vi "Cache.DUT.Read.vi"(8 "error in (no error)":errorcluster, 11 "ResultsPath":path=path "D:/svn/LineTraceSystem/SOFTWARE/logs/results") -> (0 "error out":errorcluster, 1 "Groups":i32[](array[numeric]), 2 "Results out":T1[](array[typedef]))   [LabVIEW 2016]
uses:
  Cache.TestSteps.Fglb.ResultData.ctl
  Database/ProdaNG/Controls/ProdaNG.ProcessResult.ctl
  Database/ProdaNG/Controls/ProdaNG.ProcessStepResult.ctl
  Database/ProdaNG/Controls/ProdaNG.TestStepResult.ctl
  Database/ProdaNG/Controls/ProdaNG.TestValueResult.ctl
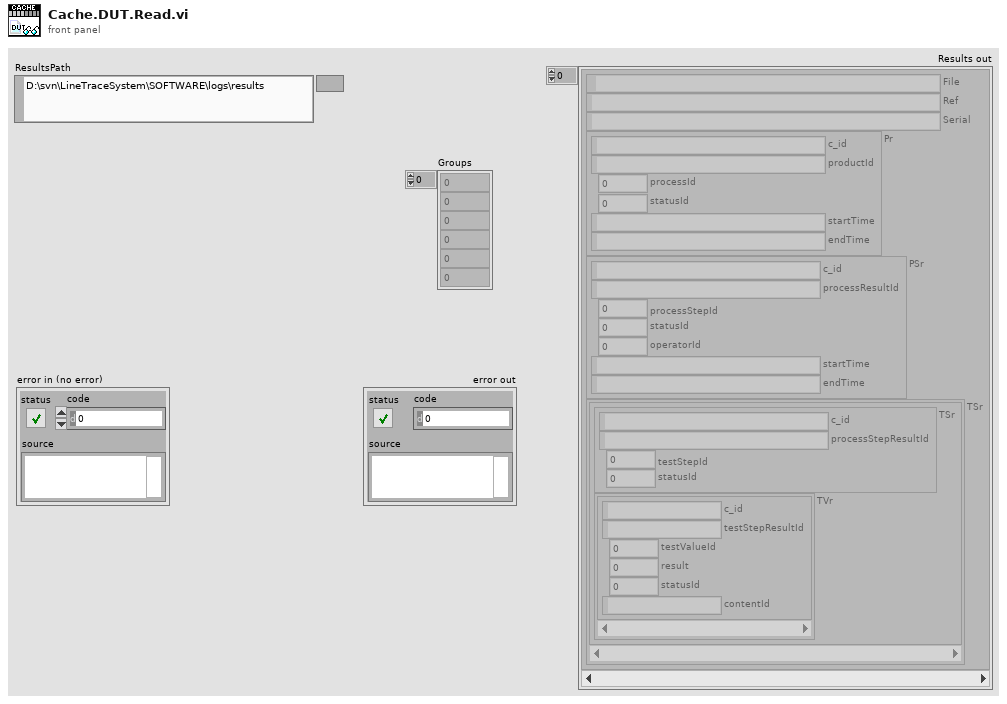
[diagram p1: front panel]
types:
  T1 = typedef "Cache.TestSteps.Fglb.ResultData.ctl" = cluster{"File":path, "Ref":string, "Serial":string, "Pr":T2, "PSr":T3, "TSr":cluster{"TSr":T4, "TVr":T5[]}[]}
  T2 = typedef "ProdaNG.ProcessResult.ctl" = cluster{"c_id":string, "productId":string, "processId":i32, "statusId":i32, "startTime":string, "endTime":string}
  T3 = typedef "ProdaNG.ProcessStepResult.ctl" = cluster{"c_id":string, "processResultId":string, "processStepId":i32, "statusId":i32, "operatorId":i32, "startTime":string, "endTime":string}
  T4 = typedef "ProdaNG.TestStepResult.ctl" = cluster{"c_id":string, "processStepResultId":string, "testStepId":i32, "statusId":i32}
  T5 = typedef "ProdaNG.TestValueResult.ctl" = cluster{"c_id":string, "testStepResultId":string, "testValueId":i32, "result":dbl, "statusId":i32, "contentId":string}
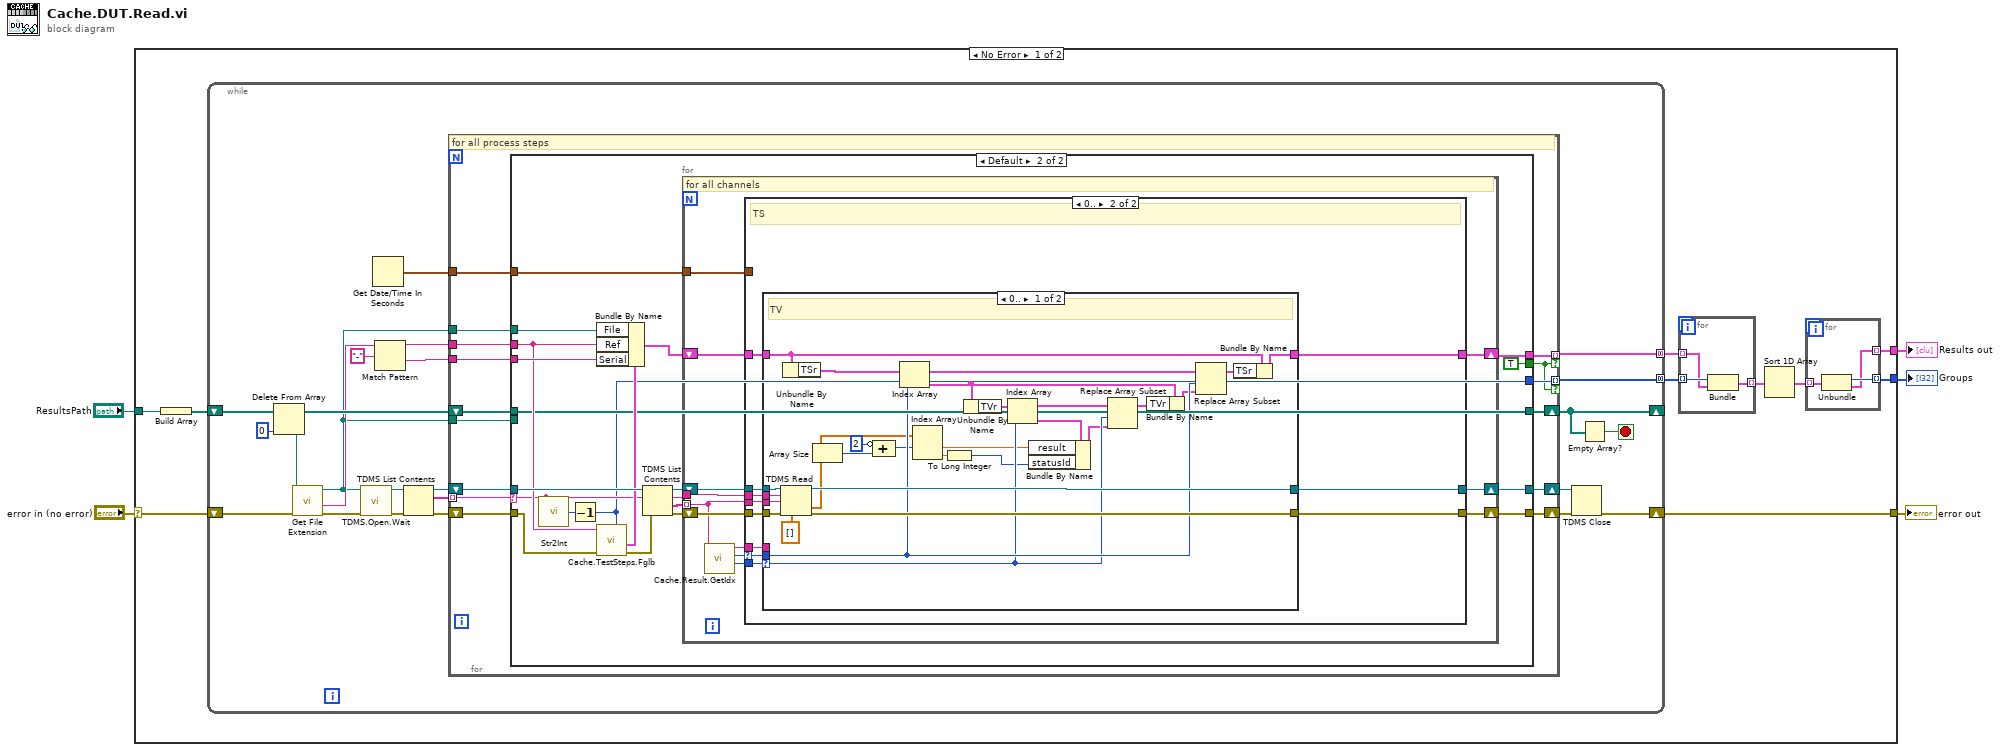
[diagram p0: block diagram]
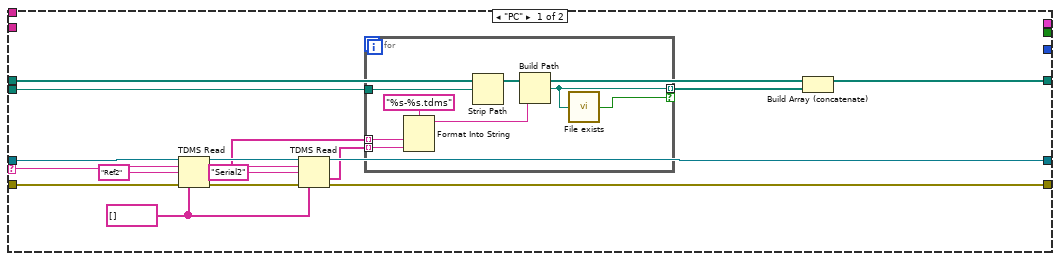
[diagram p2: hidden frame]
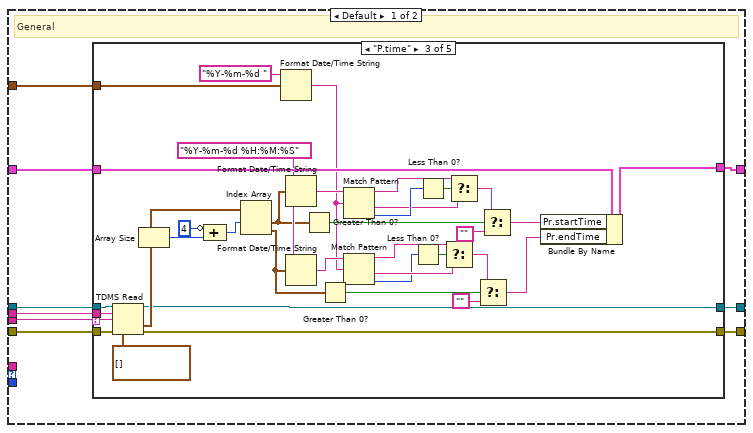
[diagram p3: hidden frame]
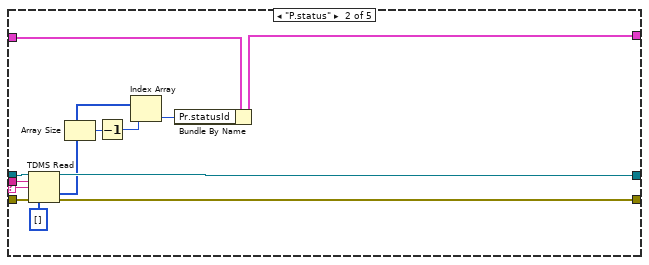
[diagram p5: hidden frame]
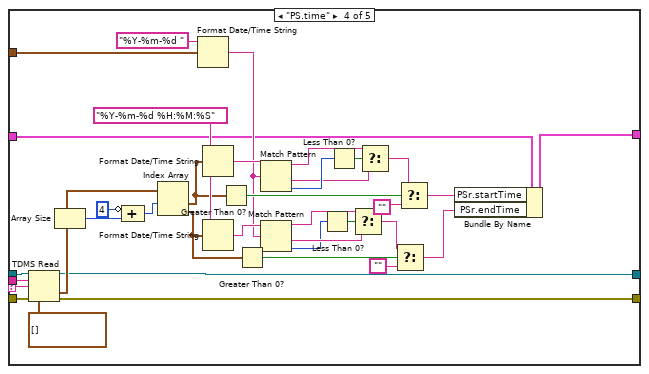
[diagram p6: hidden frame]
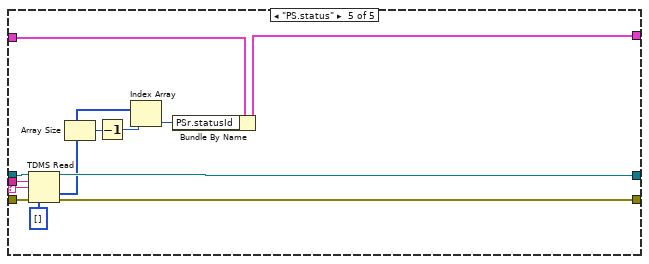
[diagram p7: hidden frame]
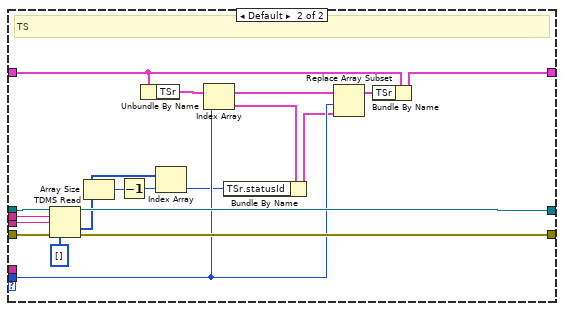
[diagram p8: hidden frame]
diagram:
  n1 = case shown="No Error" "error in (no error)" {
    selector: "error in (no error)" -> [w14 w286]
    tunnel: [w15 w286] -> w5
    tunnel: "ResultsPath" -> [w13 _]
    tunnel: [w6 _] -> w2
    tunnel: [w7 _] -> w1
    frame No Error {
      n2 = Build Array(w13) -> (w12:path[])
      n3 = while {
        tunnel: [w44] -> w11 mode=concatenating
        tunnel: [w42] -> w10 mode=concatenating
        shift-right: [w45] -> w15
        shift-left: w14 -> [w43]
        shift-right: [w25] -> _
        shift-left: w12 -> [w41]
        stop <- w24 stop-if-true
        n4 = Delete From Array(array=w41, index=0) -> (deleted portion=w27:path, array with subset deleted=w26:path[])  [unwired: 1 in]
        n5 = call <vilib>:"Get File Extension.vi"("error in (no error)"=w43, "file"=w27) -> ("error out"=w35:errorcluster, "filename without extension"=w23:string, "dup file"=w22:path)  [unwired: 5 in, 2 out]
        n6 = call "TDMS.Open.Wait.vi"("error in (no error)"=w35, "file path"=w22) -> ("error out"=w31:errorcluster, "tdms file out"=w38:refnum<k34>)  [unwired: 8 in]
        n7 = Get Date/Time In Seconds() -> (seconds since 1Jan1904=w29:timestamp)
        n8 = Match Pattern(string=w23, regular expression="-") -> (before substring=w33:string, after substring=w32:string)  [unwired: 1 in, 2 out]
        n9 = TDMS List Contents(4:w31, 7:w38) -> (0:w39:errorcluster, 2:w30:string[], 3:w40:refnum<k34>)  [unwired: 1 in, 1 out]
        n10 = for {
          shift-right: [w60] -> w37
          shift-left: w39 -> [w55]
          shift-right: [w59] -> w36
          shift-left: w40 -> [w57]
          tunnel: w30 -> [w52] mode=indexing
          tunnel: [w58] -> w44 mode=indexing if=w47
          tunnel: w33 -> [w54]
          tunnel: w32 -> [w56]
          tunnel: w29 -> [w53]
          tunnel: w22 -> [w51]
          shift-right: [w49] -> w25
          shift-left: w26 -> [w50]
          tunnel: [w48] -> w42 mode=indexing if=w47
          tunnel: w22 -> [w46]
          # "for all process steps"
          n11 = case shown="Default" w52 {
            selector: w52 -> [w75 w89]
            tunnel: [w68 w106] -> w60
            tunnel: [w67 w105] -> w59
            tunnel: [_ w104] -> w58
            tunnel: w57 -> [w76 w102]
            tunnel: w56 -> [_ w96]
            tunnel: w55 -> [w77 w95]
            tunnel: w54 -> [_ w94]
            tunnel: w53 -> [_ w93]
            tunnel: w51 -> [w66 _]
            tunnel: [_ TRUE] -> w47
            tunnel: w50 -> [w62 w90]
            tunnel: [w61 w90] -> w49
            tunnel: [_ w87] -> w48
            tunnel: w46 -> [_ w86]
            frame "PC" {
              w69 = string[] [] ("data type")
              n12 = TDMS Read(0:w76, 5:w75, 7:"Ref2" ("channel name(s) in"), 11:w77, 12:w69) -> (4:w72:refnum<k34>, 6:w70:string, 10:w64:string[], 15:w71:errorcluster)  [unwired: 3 in, 2 out]
              n13 = TDMS Read(0:w72, 5:w70, 7:"Serial2" ("channel name(s) in"), 11:w71, 12:w69) -> (4:w67:refnum<k34>, 10:w65:string[], 15:w68:errorcluster)  [unwired: 3 in, 3 out]
              n14 = for {
                tunnel: w64 -> [w85] mode=indexing
                tunnel: w66 -> [w82]
                tunnel: w65 -> [w84] mode=indexing
                tunnel: [w79] -> w63 mode=indexing if=w78
                n15 = Format Into String(format string="%s-%s.tdms", w85, w84) -> (resulting string=w80:string)  [unwired: 2 in, 1 out]
                n16 = Strip Path(path=w82) -> (stripped path=w81:path)  [unwired: 1 out]
                n17 = Build Path(base path=w81, name or relative path=w80) -> (appended path=w79:path)
                n18 = call "File exists.vi"("file path"=w79) -> ("exists?"=w78:bool)  [unwired: 4 in]
              }
              n19 = Build Array (concatenate)(w62, w63) -> (w61:path[])
            }
            frame Default {
              n20 = call "Str2Int.vi"("string"=w89) -> ("Numeric"=w88:i32)
              n21 = Decrement(x=w88) -> (x-1=w87:i32)
              n22 = call "Cache.TestSteps.Fglb.vi"("SystemIdx"=w87, "error in (no error)"=w95, "Variant"=w94) -> ("error out"=w92:errorcluster, "Result out"=w98:T1)  [unwired: 5 in, 2 out]
              n23 = Bundle By Name(cluster=w98, "File"=w86, "Ref"=w94, "Serial"=w96) -> (w97:T1)
              n24 = TDMS List Contents(4:w92, 6:w89, 7:w102) -> (0:w100:errorcluster, 1:w99:string[], 2:w103:string, 3:w101:refnum<k34>)
              n25 = for {
                tunnel: w103 -> [w109]
                shift-right: [w116] -> w105
                shift-left: w101 -> [w118]
                shift-right: [w114] -> w104
                shift-left: w97 -> [w115]
                shift-right: [w117] -> w106
                shift-left: w100 -> [w110]
                tunnel: w99 -> [w108] mode=indexing
                tunnel: w93 -> [w107]
                # "for all channels"
                n26 = call "Cache.Result.GetIdx.vi"("String"=w108) -> ("TV idx"=w112:i32, "TS idx"=w113:i32, "remaining string"=w111:string)  [unwired: 8 in]
                n27 = case shown="0.." w113 {
                  selector: w113 -> [_ w233]
                  tunnel: w112 -> [_ w232]
                  tunnel: w110 -> [w127 w241]
                  tunnel: w108 -> [w126 w240]
                  tunnel: w118 -> [w124 w239]
                  tunnel: w109 -> [w125 w238]
                  tunnel: [w123 w237] -> w117
                  tunnel: [w122 w236] -> w116
                  tunnel: w115 -> [w121 w235]
                  tunnel: [w120 w234] -> w114
                  tunnel: w111 -> [_ w231]
                  tunnel: w107 -> [w119 _]
                  frame Default {
                    # "General"
                    n28 = case shown="\"P.time\"" w126 {
                      selector: w126 -> [_ w140 w177 w214 w227]
                      tunnel: w127 -> [w128 w143 w180 w217 w230]
                      tunnel: w124 -> [w129 w142 w179 w216 w229]
                      tunnel: w125 -> [_ w141 w178 w215 w228]
                      tunnel: [w128 w139 w176 w213 w226] -> w123
                      tunnel: [w129 w138 w172 w209 w225] -> w122
                      tunnel: w121 -> [w130 w136 w171 w183 w223]
                      tunnel: [w130 w135 w174 w211 w222] -> w120
                      tunnel: w119 -> [_ _ w157 w196 _]
                      frame Default {
                      }
                      frame "P.status" {
                        n29 = TDMS Read(0:w142, 5:w141, 7:w140, 11:w143, 12:i32[] []) -> (4:w138:refnum<k34>, 10:w131:i32[], 15:w139:errorcluster)  [unwired: 3 in, 3 out]
                        n30 = Array Size(array=w131) -> (size(s)=w134:i32)
                        n31 = Decrement(x=w134) -> (x-1=w133:i32)
                        n32 = Index Array(array=w131, index=w133) -> (element=w132:i32)
                        n33 = Bundle By Name(cluster=w136, "Pr.statusId"=w132) -> (w135:T1)
                      }
                      frame "P.time" {
                        w168 = "%Y-%m-%d %H:%M:%S" ("time format string (%c)")
                        n34 = TDMS Read(0:w179, 5:w178, 7:w177, 11:w180, 12:timestamp[] []) -> (4:w172:refnum<k34>, 10:w173:timestamp[], 15:w176:errorcluster)  [unwired: 3 in, 3 out]
                        n35 = Array Size(array=w173) -> (size(s)=w170:i32)
                        n36 = Compound Arithmetic op=ADD(invert 4 ("value"), w170) -> (w169:i32)
                        n37 = Index Array(array=w173, index #1=w169) -> (element #1=w166:timestamp, element #2=w164:timestamp)  [unwired: 1 in]
                        n38 = Format Date/Time String(time format string (%c)="%Y-%m-%d ", seconds (now)=w157) -> (date/time string=w148:string)  [unwired: 1 in]
                        n39 = Format Date/Time String(time format string (%c)=w168, seconds (now)=w166) -> (date/time string=w158:string)  [unwired: 1 in]
                        n40 = Format Date/Time String(time format string (%c)=w168, seconds (now)=w164) -> (date/time string=w149:string)  [unwired: 1 in]
                        n41 = Greater Than 0?(x=w166) -> (x > 0?=w167:bool)
                        n42 = Greater Than 0?(x=w164) -> (x > 0?=w165:bool)
                        n43 = Match Pattern(string=w158, regular expression=w148) -> (before substring=w145:string, after substring=w154:string, offset past match=w156:i32)  [unwired: 1 in, 1 out]
                        n44 = Match Pattern(string=w149, regular expression=w148) -> (before substring=w146:string, after substring=w152:string, offset past match=w150:i32)  [unwired: 1 in, 1 out]
                        n45 = Less Than 0?(x=w150) -> (x < 0?=w151:bool)
                        n46 = Less Than 0?(x=w156) -> (x < 0?=w155:bool)
                        n47 = Select(t=w146, s=w151, f=w152) -> (s? t:f=w147:string)
                        n48 = Select(t=w145, s=w155, f=w154) -> (s? t:f=w153:string)
                        n49 = Select(t=w147, s=w165, f="") -> (s? t:f=w161:string)
                        n50 = Select(t=w153, s=w167, f="") -> (s? t:f=w160:string)
                        n51 = Bundle By Name(cluster=w171, "Pr.startTime"=w160, "Pr.endTime"=w161) -> (w174:T1)
                      }
                      frame "PS.time" {
                        w206 = "%Y-%m-%d %H:%M:%S" ("time format string (%c)")
                        n52 = TDMS Read(0:w216, 5:w215, 7:w214, 11:w217, 12:timestamp[] []) -> (4:w209:refnum<k34>, 10:w210:timestamp[], 15:w213:errorcluster)  [unwired: 3 in, 3 out]
                        n53 = Array Size(array=w210) -> (size(s)=w208:i32)
                        n54 = Compound Arithmetic op=ADD(invert 4 ("value"), w208) -> (w207:i32)
                        n55 = Index Array(array=w210, index #1=w207) -> (element #1=w204:timestamp, element #2=w202:timestamp)  [unwired: 1 in]
                        n56 = Format Date/Time String(time format string (%c)="%Y-%m-%d ", seconds (now)=w196) -> (date/time string=w187:string)  [unwired: 1 in]
                        n57 = Format Date/Time String(time format string (%c)=w206, seconds (now)=w204) -> (date/time string=w197:string)  [unwired: 1 in]
                        n58 = Format Date/Time String(time format string (%c)=w206, seconds (now)=w202) -> (date/time string=w188:string)  [unwired: 1 in]
                        n59 = Greater Than 0?(x=w204) -> (x > 0?=w205:bool)
                        n60 = Greater Than 0?(x=w202) -> (x > 0?=w203:bool)
                        n61 = Match Pattern(string=w197, regular expression=w187) -> (before substring=w184:string, after substring=w193:string, offset past match=w195:i32)  [unwired: 1 in, 1 out]
                        n62 = Match Pattern(string=w188, regular expression=w187) -> (before substring=w185:string, after substring=w191:string, offset past match=w189:i32)  [unwired: 1 in, 1 out]
                        n63 = Less Than 0?(x=w189) -> (x < 0?=w190:bool)
                        n64 = Less Than 0?(x=w195) -> (x < 0?=w194:bool)
                        n65 = Select(t=w185, s=w190, f=w191) -> (s? t:f=w186:string)
                        n66 = Select(t=w184, s=w194, f=w193) -> (s? t:f=w192:string)
                        n67 = Select(t=w186, s=w203, f="") -> (s? t:f=w199:string)
                        n68 = Select(t=w192, s=w205, f="") -> (s? t:f=w182:string)
                        n69 = Bundle By Name(cluster=w183, "PSr.startTime"=w182, "PSr.endTime"=w199) -> (w211:T1)
                      }
                      frame "PS.status" {
                        n70 = TDMS Read(0:w229, 5:w228, 7:w227, 11:w230, 12:i32[] []) -> (4:w225:refnum<k34>, 10:w218:i32[], 15:w226:errorcluster)  [unwired: 3 in, 3 out]
                        n71 = Array Size(array=w218) -> (size(s)=w221:i32)
                        n72 = Decrement(x=w221) -> (x-1=w220:i32)
                        n73 = Index Array(array=w218, index=w220) -> (element=w219:i32)
                        n74 = Bundle By Name(cluster=w223, "PSr.statusId"=w219) -> (w222:T1)
                      }
                    }
                  }
                  frame 0.. {
                    # "TS"
                    n75 = case shown="0.." w232 {
                      selector: w232 -> [w258 _]
                      tunnel: w241 -> [w265 w283]
                      tunnel: w240 -> [w262 w280]
                      tunnel: w239 -> [w264 w282]
                      tunnel: w238 -> [w263 w281]
                      tunnel: [w260 w278] -> w237
                      tunnel: [w261 w279] -> w236
                      tunnel: w235 -> [w266 w284]
                      tunnel: [w267 w285] -> w234
                      tunnel: w233 -> [w259 w277]
                      tunnel: w231 -> [_ _]
                      frame 0.. {
                        # "TV"
                        n76 = TDMS Read(0:w264, 5:w263, 7:w262, 11:w265, 12:dbl[] []) -> (4:w261:refnum<k34>, 10:w246:dbl[], 15:w260:errorcluster)  [unwired: 3 in, 3 out]
                        n77 = Unbundle By Name(w266) -> ("TSr"=w251:cluster{"TSr":T4, "TVr":T5[]}[])
                        n78 = Array Size(array=w246) -> (size(s)=w245:i32)
                        n79 = Compound Arithmetic op=ADD(invert 2 ("value"), w245) -> (w244:i32)
                        n80 = Index Array(array=w251, index=w259) -> (element=w252:cluster{"TSr":T4, "TVr":T5[]})
                        n81 = Index Array(array=w246, index #1=w244) -> (element #1=w248:dbl, element #2=w247:dbl)  [unwired: 1 in]
                        n82 = To Long Integer(number=w247) -> (32bit integer=w243:i32)
                        n83 = Unbundle By Name(w252) -> ("TVr"=w255:T5[])
                        n84 = Index Array(array=w255, index=w258) -> (element=w256:T5)
                        n85 = Bundle By Name(cluster=w256, "result"=w248, "statusId"=w243) -> (w254:T5)
                        n86 = Replace Array Subset(array=w255, new element=w254, index=w258) -> (w253:T5[])
                        n87 = Bundle By Name(cluster=w252, "TVr"=w253) -> (w249:cluster{"TSr":T4, "TVr":T5[]})
                        n88 = Replace Array Subset(array=w251, new element=w249, index=w259) -> (w250:cluster{"TSr":T4, "TVr":T5[]}[])
                        n89 = Bundle By Name(cluster=w266, "TSr"=w250) -> (w267:T1)
                      }
                      frame Default {
                        # "TS"
                        n90 = TDMS Read(0:w282, 5:w281, 7:w280, 11:w283, 12:i32[] []) -> (4:w279:refnum<k34>, 10:w270:i32[], 15:w278:errorcluster)  [unwired: 3 in, 3 out]
                        n91 = Array Size(array=w270) -> (size(s)=w269:i32)
                        n92 = Decrement(x=w269) -> (x-1=w268:i32)
                        n93 = Unbundle By Name(w284) -> ("TSr"=w274:cluster{"TSr":T4, "TVr":T5[]}[])
                        n94 = Index Array(array=w270, index=w268) -> (element=w271:i32)
                        n95 = Index Array(array=w274, index=w277) -> (element=w275:cluster{"TSr":T4, "TVr":T5[]})
                        n96 = Bundle By Name(cluster=w275, "TSr.statusId"=w271) -> (w272:cluster{"TSr":T4, "TVr":T5[]})
                        n97 = Replace Array Subset(array=w274, new element=w272, index=w277) -> (w273:cluster{"TSr":T4, "TVr":T5[]}[])
                        n98 = Bundle By Name(cluster=w284, "TSr"=w273) -> (w285:T1)
                      }
                    }
                  }
                }
              }
            }
          }
        }
        n99 = TDMS Close(8:w37, 11:w36) -> (0:w45:errorcluster)  [unwired: 1 out]
        n100 = Empty Array?(array=w25) -> (empty?=w24:bool)
      }
      n101 = for {
        tunnel: w11 -> [w20] mode=indexing
        tunnel: w10 -> [w21] mode=indexing
        tunnel: [w19] -> w9 mode=indexing
        n102 = Bundle(w21, "Result out"=w20) -> (w19:cluster{i32, "Result out":T1})  [unwired: 1 in]
      }
      n103 = Sort 1D Array(array=w9) -> (sorted array=w8:cluster{i32, "Result out":T1}[])
      n104 = for {
        tunnel: w8 -> [w18] mode=indexing
        tunnel: [w17] -> w7 mode=indexing
        tunnel: [w16] -> w6 mode=indexing
        n105 = Unbundle(w18) -> (w17:i32, "Result out"=w16:T1)
      }
    }
    frame Error {
    }
  }
  "error out" <- w5
  "Results out" <- w2
  "Groups" <- w1
